vi "LinearPlntInvFF_GetUff.vi"(11 "Linear Plnt Inversion FF":T2) -> (3 "Uff":T1)   [LabVIEW 2019, in "Trajectory_Library.lvlib"]
doc: "Returns the previously calculated feedforward as an input vector.\n\nInputs:\n - LinearPlntInversionFF -- system data cluster\n\nOutputs:\n - Uff -- The calculated feedforward."
uses:
  Trajectory_Library.lvlib
  LINEAR_PLANT_INV_FF.ctl
  <vilib>/Analysis/Matrix/Datatypes/RealMatrix.ctl
  <vilib>/Analysis/Matrix/NI_Matrix.lvlib
panel:
  # "<States,1>"
  # "<Inputs,1>"
  # "<States,Inputs>"
  # "<States,States>"
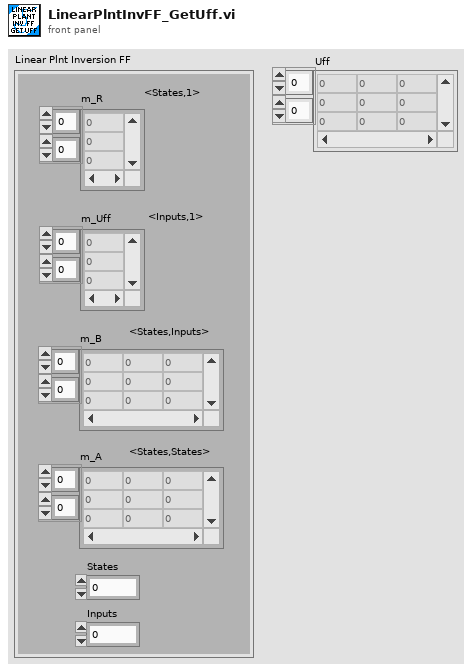
[diagram p1: front panel]
types:
  T1 = typedef "NI_Matrix.lvlib/RealMatrix.ctl" = dbl[][]
  T2 = typedef "Trajectory_Library.lvlib/LINEAR_PLANT_INV_FF.ctl" = cluster{"m_R":T1, "m_Uff":T1, "m_B":T1, "m_A":T1, "States":i32, "Inputs":i32}
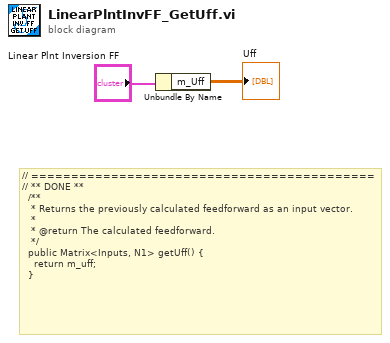
[diagram p0: block diagram]
diagram:
  # "// ===========================================\n// ** DONE **\n  /**\n   * Returns the previously calculated feedforward as an input vector.\n   *\n   * @return The calculated feedforward.\n   */\n  public Matrix<Inputs, N1> getUff() {\n    return m_uff;\n  }"
  n1 = Unbundle By Name("Linear Plnt Inversion FF") -> ("m_Uff"=→"Uff":T1)
